vi "Do.vi"(8 "Error In":errorcluster, 10 "Actor in":refnum<class "Actor.lvclass">, 11 "LNA Connection Status Msg":refnum<class "LNA Connection Status Msg.lvclass">) -> (0 "Error Out":errorcluster, 2 "Actor out":refnum<class "Actor.lvclass">)   [LabVIEW 2016, in "TestLNA.lvlib" / "LNA Connection Status Msg.lvclass"]
doc: "(<B>Filename</B>: Actor Framework.lvlib:Message.lvclass:Do.vi)\n\nDefines what a message does when it is received by an actor. Generally, a message instructs an actor to invoke one of its methods. By default, this method does nothing. A child class must override it to define behavior. Create a child class by using the Actor Framework Message Maker dialog box."
uses:
  LNA Connection Status Msg.lvclass
  C:/Program Files (x86)/National Instruments/LabVIEW 2016/vi.lib/NI/Actors/Linked Network Actor/Linked Network Actor Messages/LNA Connection Status Msg/LNA Connection Status Msg.lvclass
  <vilib>/ActorFramework/Actor/Actor.lvclass
  TestLNA.lvclass
  C:/Program Files (x86)/National Instruments/LabVIEW 2016/vi.lib/ActorFramework/Actor/Actor.lvclass
  <vilib>/NI/Actors/Linked Network Actor/Linked Network Actor Messages/LNA Connection Status Msg/LNA Connection Status Msg.lvclass/LNA Connection Status Msg.ctl
  TestLNA.lvclass/TestLNA.ctl
  <vilib>/NI/Actors/Linked Network Actor/Linked Network Actor Messages/LNA Connection Status Msg/LNA Connection Status Msg.lvclass
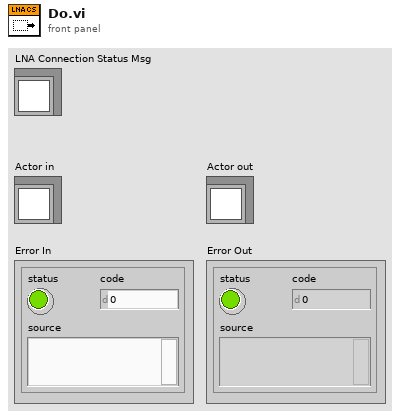
[diagram p1: front panel]
types:
  T1 = cluster{"Name":string, "Writer":bool, "Reader":bool}
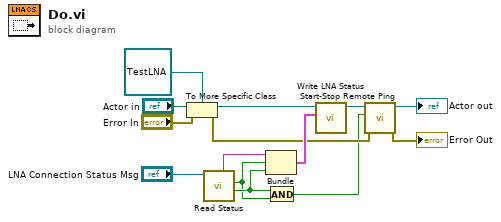
[diagram p0: block diagram]
diagram:
  n1 = To More Specific Class(target class=refnum<class "TestLNA.lvclass"> refnum ("Test LNA.lvlib:Test LNA.lvclass"), reference="Actor in", error in="Error In") -> (specific class reference=w12:refnum<class "TestLNA.lvclass">, error out=w5:errorcluster)
  n2 = call <vilib>:"Read Status.vi"("Update Status Msg in"="LNA Connection Status Msg") -> ("Reader"=w3:bool, "Writer"=w2:bool, "Name"=w9:string)  [unwired: 7 in, 1 out]
  n3 = Bundle("Name"=w9, "Writer"=w2, "Reader"=w3) -> (w8:T1)  [unwired: 1 in]
  n4 = And(x=w3, y=w2) -> (x .and. y?=w1:bool)
  n5 = call "Write LNA Status.vi"("LNA Status"=w8, "Test LNA in"=w12) -> ("Test LNA out"=w7:refnum<class "TestLNA.lvclass">)  [unwired: 9 in]
  n6 = call "Start-Stop Remote Ping.vi"("Error In"=w5, "Start Remote Ping"=w1, "Test LNA in"=w7) -> ("Error Out"=→"Error Out":errorcluster, "Test LNA out"=→"Actor out":refnum<class "TestLNA.lvclass">)  [unwired: 7 in]
